vi "arduino digital pin on off.vi"(9 "Arduino VISA in":refnum<visa-resource-name>="Arduino", 11 "pin states 2-13":bool[](array[boolean])) -> ()   [LabVIEW 2020]
uses:
  <vilib>/LabVIEW Interface for Arduino/Type Defs/Pin Mode.ctl
  <vilib>/LabVIEW Interface for Arduino/LabVIEW Interface for Arduino.lvlib
panel:
  # "5"
  # "12"
  # "5-7=TTL\n12=LED"
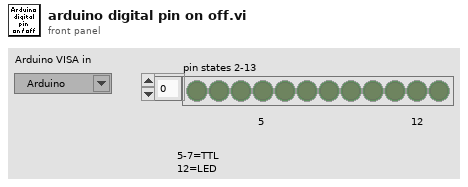
[diagram p1: front panel]
types:
  T1 = typedef "LabVIEW Interface for Arduino.lvlib/Arduino Resource.ctl" = cluster{"VISA resource":refnum<visa-resource-name>, "Board Type":T2, "Connection Type":enum8{"USB / Serial"}, "Bytes Per Packet (15)":u8}
  T2 = typedef "LabVIEW Interface for Arduino.lvlib/Board Type.ctl" = enum16{"Uno", "Dimuelanove w/Atmega 328", "Mega 2560"}
  T3 = typedef "LabVIEW Interface for Arduino.lvlib/Pin Mode.ctl" = enum8{"Input", "Output"}
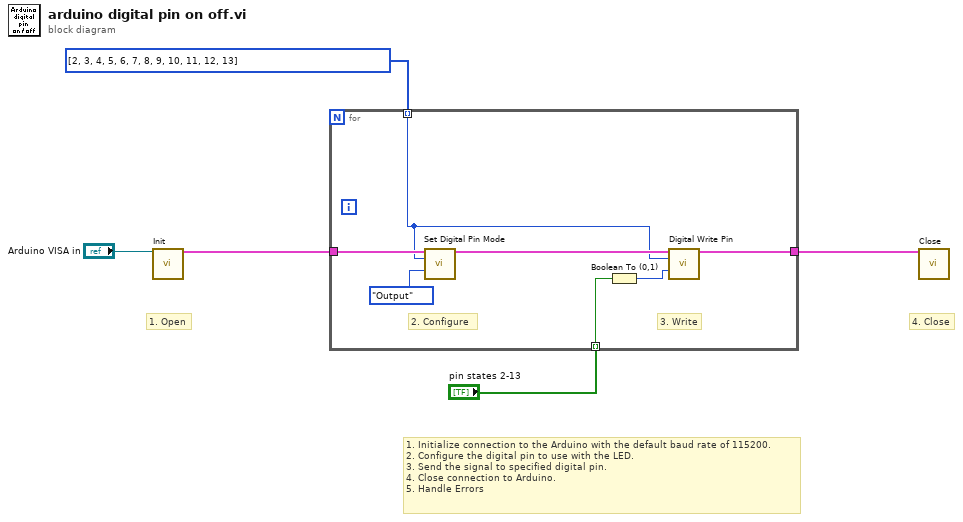
[diagram p0: block diagram]
diagram:
  # "4. Close"
  # "1. Open"
  # "1. Initialize connection to the Arduino with the default baud rate of 115200.\n2. Configure the digital pin to use with the LED.\n3. Send the signal to specified digital pin.\n4. Close connection to Arduino.\n5. Handle Errors"
  n1 = call <vilib>:"Init.vi"("VISA resource"="Arduino VISA in") -> ("Arduino Resource"=w4:T1)  [unwired: 17 in, 1 out]
  n2 = for {
    tunnel: w4 -> [w11]
    tunnel: [w12] -> w5
    tunnel: i32[] [2, 3, 4, 5, 6, 7, 8, 9, 10, 11, 12, 13] ("x+y") -> [w7] mode=indexing
    tunnel: "pin states 2-13" -> [w6] mode=indexing
    # "3. Write"
    # "2. Configure"
    n3 = call <vilib>:"Set Digital Pin Mode.vi"("Arduino Resource"=w11, "Digital I/O Pin"=w7, "Pin Mode (Input)"=Pin_Mode."Output") -> ("Arduino Resource"=w10:T1)  [unwired: 11 in, 1 out]
    n4 = Boolean To (0,1)(Boolean=w6) -> (0, 1=w8:i16)
    n5 = call <vilib>:"Digital Write Pin.vi"("Arduino Resource"=w10, "Digital I/O Pin (0)"=w7, "Value (0)"=w8) -> ("Arduino Resource"=w12:T1)  [unwired: 11 in, 1 out]
  }
  n6 = call <vilib>:"Close.vi"("Arduino Resource"=w5) -> ()  [unwired: 14 in, 1 out]
